vi "Register Service.vi"(8 "error in (no error)":errorcluster, 10 "Service":refnum<class "Service.lvclass">, 11 "Service Container in":refnum<class "Service Container.lvclass">) -> (0 "error out":errorcluster, 3 "Service Container out":refnum<class "Service Container.lvclass">)   [LabVIEW 2020, in "Vecto.lvlib" / "Service Container.lvclass"]
uses:
  Service Container.lvclass
  Service/Service.lvclass
  Service Container.lvclass/Service Container.ctl
  <vilib>/Utility/miscctls.llb/LVMapReplaceAction.ctl
  <vilib>/Utility/error.llb/Error Cluster From Error Code.vi
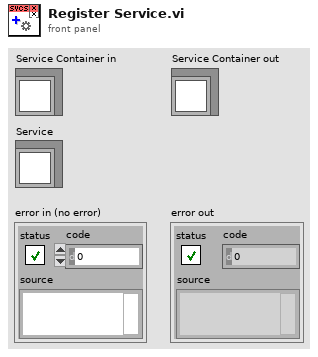
[diagram p1: front panel]
types:
  T1 = typedef "LVMapReplaceAction.ctl" = enum32{"Modify Entry only if found", "Add or Modify Entry", "Delete Entry"}
  T2 = typedef "Vecto.lvlib/Service Container.lvclass/Services.ctl" = map{string, map{string, refnum<class "Service.lvclass">}}
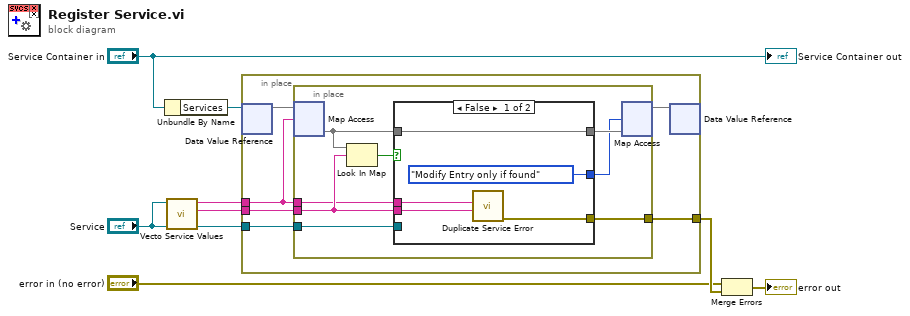
[diagram p0: block diagram]
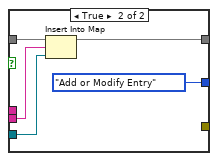
[diagram p2: hidden frame]
diagram:
  n1 = Unbundle By Name("Service Container in") -> ("Services"=w7:refnum<data-value>)
  n2 = call "Vecto Service Values.vi"("Service in"="Service") -> ("ID"=w5:string, "Type"=w6:string)  [unwired: 9 in]
  n3 = in-place {
    in-place-border: w6 -> [w10]
    in-place-border: w5 -> [w13]
    in-place-border: "Service" -> [w11]
    in-place-border: [w9] -> w3
    n4 = in-place-dvr #1(w7) -> (w14:T2)  [unwired: 1 out]
    n5 = in-place {
      in-place-border: w13 -> [w20]
      in-place-border: w11 -> [w19]
      in-place-border: w10 -> [w16]
      in-place-border: [w15] -> w9
      n6 = in-place-map #2(w14, w10) -> (w21:map{string, refnum<class "Service.lvclass">})  [unwired: 1 in, 1 out]
      n7 = Look In Map(map=w21, key=w20) -> (key not found?=w22:bool)  [unwired: 1 in, 1 out]
      n8 = case shown="False" w22 {
        tunnel: w21 -> [w26 w32]
        tunnel: w20 -> [w24 w31]
        tunnel: w19 -> [_ w30]
        tunnel: [w26 w29] -> w18
        tunnel: [LVMapReplaceAction."Modify Entry only if found" ("action") LVMapReplaceAction."Add or Modify Entry" ("action")] -> w17
        tunnel: w16 -> [w25 _]
        tunnel: [w23 _] -> w15
        frame False {
          n9 = call "Duplicate Service Error.vi"("ID"=w24, "Type"=w25) -> ("error out"=w23:errorcluster)  [unwired: 9 in]
        }
        frame True {
          n10 = Insert Into Map(map in=w32, key=w31, value=w30) -> (map out=w29:map{string, refnum<class "Service.lvclass">})  [unwired: 2 out]
        }
      }
      n11 = in-place-map #2(w18, w17) -> (w12:T2)  [unwired: 2 out]
    }
    n12 = in-place-dvr #1(w12) -> ()  [unwired: 2 out]
  }
  n13 = Merge Errors("error in (no error)", w3) -> (→"error out":errorcluster)
  "Service Container out" <- "Service Container in"
